vi "test TCX read (installed 71).vi"() -> ()   [LabVIEW 2011] (continued)
ers><DistanceMeters>9789.869</DistanceMeters><Cadence>71</Cadence><Extensions><TPX xmlns=\"http://www.garmin.com/xmlschemas/ActivityExtension/v2\"><Watts>262</Watts></TPX></Extensions></Trackpoint><Trackpoint><Time>2008-03-03T14:06:44Z</Time><Position><LatitudeDegrees>35.860413</LatitudeDegrees><LongitudeDegrees>-78.885609</LongitudeDegrees></Position><AltitudeMeters>95.788</AltitudeMeters><DistanceMeters>9797.562</DistanceMeters><Cadence>71</Cadence><Extensions><TPX xmlns=\"http://www.garmin.com/xmlschemas/ActivityExtension/v2\"><Watts>280</Watts></TPX></Extensions></Trackpoint><Trackpoint><Time>2008-03-03T14:06:45Z</Time><Position><LatitudeDegrees>35.860470</LatitudeDegrees><LongitudeDegrees>-78.885560</LongitudeDegrees></Position><AltitudeMeters>95.788</AltitudeMeters><DistanceMeters>9805.292</DistanceMeters><Cadence>71</Cadence><Extensions><TPX xmlns=\"http://www.garmin.com/xmlschemas/ActivityExtension/v2\"><Watts>243</Watts></TPX></Extensions></Trackpoint><Trackpoint><Time>2008-03-03T14:06:46Z</Time><Position><LatitudeDegrees>35.860528</LatitudeDegrees><LongitudeDegrees>-78.885512</LongitudeDegrees></Position><AltitudeMeters>96.269</AltitudeMeters><DistanceMeters>9813.017</DistanceMeters><Cadence>71</Cadence><Extensions><TPX xmlns=\"http://www.garmin.com/xmlschemas/ActivityExtension/v2\"><Watts>199</Watts></TPX></Extensions></Trackpoint><Trackpoint><Time>2008-03-03T14:06:47Z</Time><Position><LatitudeDegrees>35.860585</LatitudeDegrees><LongitudeDegrees>-78.885464</LongitudeDegrees></Position><AltitudeMeters>96.269</AltitudeMeters><DistanceMeters>9820.704</DistanceMeters><Cadence>71</Cadence><Extensions><TPX xmlns=\"http://www.garmin.com/xmlschemas/ActivityExtension/v2\"><Watts>198</Watts></TPX></Extensions></Trackpoint><Trackpoint><Time>2008-03-03T14:06:48Z</Time><Position><LatitudeDegrees>35.860642</LatitudeDegrees><LongitudeDegrees>-78.885415</LongitudeDegrees></Position><AltitudeMeters>96.269</AltitudeMeters><DistanceMeters>9828.424</DistanceMeters><Cadence>71</Cadence><Extensions><TPX xmlns=\"http://www.garmin.com/xmlschemas/ActivityExtension/v2\"><Watts>210</Watts></TPX></Extensions></Trackpoint><Trackpoint><Time>2008-03-03T14:06:49Z</Time><Position><LatitudeDegrees>35.860698</LatitudeDegrees><LongitudeDegrees>-78.885365</LongitudeDegrees></Position><AltitudeMeters>96.269</AltitudeMeters><DistanceMeters>9836.081</DistanceMeters><Cadence>71</Cadence><Extensions><TPX xmlns=\"http://www.garmin.com/xmlschemas/ActivityExtension/v2\"><Watts>211</Watts></TPX></Extensions></Trackpoint><Trackpoint><Time>2008-03-03T14:06:50Z</Time><Position><LatitudeDegrees>35.860754</LatitudeDegrees><LongitudeDegrees>-78.885315</LongitudeDegrees></Position><AltitudeMeters>96.269</AltitudeMeters><DistanceMeters>9843.739</DistanceMeters><Cadence>71</Cadence><Extensions><TPX xmlns=\"http://www.garmin.com/xmlschemas/ActivityExtension/v2\"><Watts>219</Watts></TPX></Extensions></Trackpoint><Trackpoint><Time>2008-03-03T14:06:51Z</Time><Position><LatitudeDegrees>35.860809</LatitudeDegrees><LongitudeDegrees>-78.885264</LongitudeDegrees></Position><AltitudeMeters>96.750</AltitudeMeters><DistanceMeters>9851.446</DistanceMeters><Cadence>71</Cadence><Extensions><TPX xmlns=\"http://www.garmin.com/xmlschemas/ActivityExtension/v2\"><Watts>217</Watts></TPX></Extensions></Trackpoint><Trackpoint><Time>2008-03-03T14:06:52Z</Time><Position><LatitudeDegrees>35.860865</LatitudeDegrees><LongitudeDegrees>-78.885214</LongitudeDegrees></Position><AltitudeMeters>97.230</AltitudeMeters><DistanceMeters>9859.071</DistanceMeters><Cadence>70</Cadence><Extensions><TPX xmlns=\"http://www.garmin.com/xmlschemas/ActivityExtension/v2\"><Watts>214</Watts></TPX></Extensions></Trackpoint><Trackpoint><Time>2008-03-03T14:06:53Z</Time><Position><LatitudeDegrees>35.860919</LatitudeDegrees><LongitudeDegrees>-78.885164</LongitudeDegrees></Position><AltitudeMeters>97.230</AltitudeMeters><DistanceMeters>9866.535</DistanceMeters><Cadence>67</Cadence><Extensions><TPX xmlns=\"http://www.garmin.com/xmlschemas/ActivityExtension/v2\"><Watts>220</Watts></TPX></Extensions></Trackpoint><Trackpoint><Time>2008-03-03T14:06:54Z</Time><Position><LatitudeDegrees>35.860975</LatitudeDegrees><LongitudeDegrees>-78.885114</LongitudeDegrees></Position><AltitudeMeters>97.230</AltitudeMeters><DistanceMeters>9874.188</DistanceMeters><Cadence>67</Cadence><Extensions><TPX xmlns=\"http://www.garmin.com/xmlschemas/ActivityExtension/v2\"><Watts>221</Watts></TPX></Extensions></Trackpoint><Trackpoint><Time>2008-03-03T14:06:55Z</Time><Position><LatitudeDegrees>35.861031</LatitudeDegrees><LongitudeDegrees>-78.885064</LongitudeDegrees></Position><AltitudeMeters>97.230</AltitudeMeters><DistanceMeters>9881.928</DistanceMeters><Cadence>69</Cadence><Extensions><TPX xmlns=\"http://www.garmin.com/xmlschemas/ActivityExtension/v2\"><Watts>245</Watts></TPX></Extensions></Trackpoint><Trackpoint><Time>2008-03-03T14:06:56Z</Time><Position><LatitudeDegrees>35.861087</LatitudeDegrees><LongitudeDegrees>-78.885015</LongitudeDegrees></Position><AltitudeMeters>96.750</AltitudeMeters><DistanceMeters>9889.609</DistanceMeters><Cadence>71</Cadence><Extensions><TPX xmlns=\"http://www.garmin.com/xmlschemas/ActivityExtension/v2\"><Watts>398</Watts></TPX></Extensions></Trackpoint><Trackpoint><Time>2008-03-03T14:06:57Z</Time><Position><LatitudeDegrees>35.861144</LatitudeDegrees><LongitudeDegrees>-78.884964</LongitudeDegrees></Position><AltitudeMeters>97.711</AltitudeMeters><DistanceMeters>9897.438</DistanceMeters><Cadence>71</Cadence><Extensions><TPX xmlns=\"http://www.garmin.com/xmlschemas/ActivityExtension/v2\"><Watts>421</Watts></TPX></Extensions></Trackpoint><Trackpoint><Time>2008-03-03T14:06:58Z</Time><Position><LatitudeDegrees>35.861201</LatitudeDegrees><LongitudeDegrees>-78.884911</LongitudeDegrees></Position><AltitudeMeters>98.192</AltitudeMeters><DistanceMeters>9905.341</DistanceMeters><Cadence>72</Cadence><Extensions><TPX xmlns=\"http://www.garmin.com/xmlschemas/ActivityExtension/v2\"><Watts>420</Watts></TPX></Extensions></Trackpoint><Trackpoint><Time>2008-03-03T14:06:59Z</Time><Position><LatitudeDegrees>35.861256</LatitudeDegrees><LongitudeDegrees>-78.884860</LongitudeDegrees></Position><AltitudeMeters>98.192</AltitudeMeters><DistanceMeters>9912.980</DistanceMeters><Cadence>71</Cadence><Extensions><TPX xmlns=\"http://www.garmin.com/xmlschemas/ActivityExtension/v2\"><Watts>419</Watts></TPX></Extensions></Trackpoint><Trackpoint><Time>2008-03-03T14:07:00Z</Time><Position><LatitudeDegrees>35.861312</LatitudeDegrees><LongitudeDegrees>-78.884809</LongitudeDegrees></Position><AltitudeMeters>98.672</AltitudeMeters><DistanceMeters>9920.728</DistanceMeters><Cadence>70</Cadence><Extensions><TPX xmlns=\"http://www.garmin.com/xmlschemas/ActivityExtension/v2\"><Watts>406</Watts></TPX></Extensions></Trackpoint><Trackpoint><Time>2008-03-03T14:07:01Z</Time><Position><LatitudeDegrees>35.861368</LatitudeDegrees><LongitudeDegrees>-78.884761</LongitudeDegrees></Position><AltitudeMeters>99.153</AltitudeMeters><DistanceMeters>9928.274</DistanceMeters><Cadence>70</Cadence><Extensions><TPX xmlns=\"http://www.garmin.com/xmlschemas/ActivityExtension/v2\"><Watts>406</Watts></TPX></Extensions></Trackpoint><Trackpoint><Time>2008-03-03T14:07:02Z</Time><Position><LatitudeDegrees>35.861424</LatitudeDegrees><LongitudeDegrees>-78.884713</LongitudeDegrees></Position><AltitudeMeters>99.634</AltitudeMeters><DistanceMeters>9935.836</DistanceMeters><Cadence>70</Cadence><Extensions><TPX xmlns=\"http://www.garmin.com/xmlschemas/ActivityExtension/v2\"><Watts>390</Watts></TPX></Extensions></Trackpoint><Trackpoint><Time>2008-03-03T14:07:03Z</Time><Position><LatitudeDegrees>35.861481</LatitudeDegrees><LongitudeDegrees>-78.884664</LongitudeDegrees></Position><AltitudeMeters>100.115</AltitudeMeters><DistanceMeters>9943.662</DistanceMeters><Cadence>69</Cadence><Extensions><TPX xmlns=\"http://www.garmin.com/xmlschemas/ActivityExtension/v2\"><Watts>387</Watts></TPX></Extensions></Trackpoint><Trackpoint><Time>2008-03-03T14:07:04Z</Time><Position><LatitudeDegrees>35.861538</LatitudeDegrees><LongitudeDegrees>-78.884615</LongitudeDegrees></Position><AltitudeMeters>100.115</AltitudeMeters><DistanceMeters>9951.247</DistanceMeters><Cadence>69</Cadence><Extensions><TPX xmlns=\"http://www.garmin.com/xmlschemas/ActivityExtension/v2\"><Watts>379</Watts></TPX></Extensions></Trackpoint><Trackpoint><Time>2008-03-03T14:07:05Z</Time><Position><LatitudeDegrees>35.861592</LatitudeDegrees><LongitudeDegrees>-78.884566</LongitudeDegrees></Position><AltitudeMeters>100.115</AltitudeMeters><DistanceMeters>9958.741</DistanceMeters><Cadence>70</Cadence><Extensions><TPX xmlns=\"http://www.garmin.com/xmlschemas/ActivityExtension/v2\"><Watts>367</Watts></TPX></Extensions></Trackpoint><Trackpoint><Time>2008-03-03T14:07:06Z</Time><Position><LatitudeDegrees>35.861647</LatitudeDegrees><LongitudeDegrees>-78.884516</LongitudeDegrees></Position><AltitudeMeters>100.595</AltitudeMeters><DistanceMeters>9966.347</DistanceMeters><Cadence>70</Cadence><Extensions><TPX xmlns=\"http://www.garmin.com/xmlschemas/ActivityExtension/v2\"><Watts>366</Watts></TPX></Extensions></Trackpoint><Trackpoint><Time>2008-03-03T14:07:07Z</Time><Position><LatitudeDegrees>35.861704</LatitudeDegrees><LongitudeDegrees>-78.884469</LongitudeDegrees></Position><AltitudeMeters>100.115</AltitudeMeters><DistanceMeters>9973.955</DistanceMeters><Cadence>72</Cadence><Extensions><TPX xmlns=\"http://www.garmin.com/xmlschemas/ActivityExtension/v2\"><Watts>375</Watts></TPX></Extensions></Trackpoint><Trackpoint><Time>2008-03-03T14:07:08Z</Time><Position><LatitudeDegrees>35.861765</LatitudeDegrees><LongitudeDegrees>-78.884424</LongitudeDegrees></Position><AltitudeMeters>100.595</AltitudeMeters><DistanceMeters>9981.838</DistanceMeters><Cadence>75</Cadence><Extensions><TPX xmlns=\"http://www.garmin.com/xmlschemas/ActivityExtension/v2\"><Watts>374</Watts></TPX></Extensions></Trackpoint><Trackpoint><Time>2008-03-03T14:07:09Z</Time><Position><LatitudeDegrees>35.861824</LatitudeDegrees><LongitudeDegrees>-78.884382</LongitudeDegrees></Position><AltitudeMeters>101.076</AltitudeMeters><DistanceMeters>9989.431</DistanceMeters><Cadence>73</Cadence><Extensions><TPX xmlns=\"http://www.garmin.com/xmlschemas/ActivityExtension/v2\"><Watts>355</Watts></TPX></Extensions></Trackpoint><Trackpoint><Time>2008-03-03T14:07:10Z</Time><Position><LatitudeDegrees>35.861884</LatitudeDegrees><LongitudeDegrees>-78.884341</LongitudeDegrees></Position><AltitudeMeters>101.076</AltitudeMeters><DistanceMeters>9997.033</DistanceMeters><Cadence>73</Cadence><Extensions><TPX xmlns=\"http://www.garmin.com/xmlschemas/ActivityExtension/v2\"><Watts>269</Watts></TPX></Extensions></Trackpoint><Trackpoint><Time>2008-03-03T14:07:11Z</Time><Position><LatitudeDegrees>35.861944</LatitudeDegrees><LongitudeDegrees>-78.884299</LongitudeDegrees></Position><AltitudeMeters>101.076</AltitudeMeters><DistanceMeters>10004.695</DistanceMeters><Cadence>73</Cadence><Extensions><TPX xmlns=\"http://www.garmin.com/xmlschemas/ActivityExtension/v2\"><Watts>270</Watts></TPX></Extensions></Trackpoint><Trackpoint><Time>2008-03-03T14:07:12Z</Time><Position><LatitudeDegrees>35.862005</LatitudeDegrees><LongitudeDegrees>-78.884257</LongitudeDegrees></Position><AltitudeMeters>101.076</AltitudeMeters><DistanceMeters>10012.445</DistanceMeters><Cadence>73</Cadence><Extensions><TPX xmlns=\"http://www.garmin.com/xmlschemas/ActivityExtension/v2\"><Watts>213</Watts></TPX></Extensions></Trackpoint><Trackpoint><Time>2008-03-03T14:07:13Z</Time><Position><LatitudeDegrees>35.862067</LatitudeDegrees><LongitudeDegrees>-78.884216</LongitudeDegrees></Position><AltitudeMeters>101.556</AltitudeMeters><DistanceMeters>10020.231</DistanceMeters><Cadence>73</Cadence><Extensions><TPX xmlns=\"http://www.garmin.com/xmlschemas/ActivityExtension/v2\"><Watts>227</Watts></TPX></Extensions></Trackpoint><Trackpoint><Time>2008-03-03T14:07:14Z</Time><Position><LatitudeDegrees>35.862130</LatitudeDegrees><LongitudeDegrees>-78.884177</LongitudeDegrees></Position><AltitudeMeters>101.556</AltitudeMeters><DistanceMeters>10028.093</DistanceMeters><Cadence>73</Cadence><Extensions><TPX xmlns=\"http://www.garmin.com/xmlschemas/ActivityExtension/v2\"><Watts>227</Watts></TPX></Extensions></Trackpoint><Trackpoint><Time>2008-03-03T14:07:15Z</Time><Position><LatitudeDegrees>35.862193</LatitudeDegrees><LongitudeDegrees>-78.884138</LongitudeDegrees></Position><AltitudeMeters>101.556</AltitudeMeters><DistanceMeters>10035.955</DistanceMeters><Cadence>73</Cadence><Extensions><TPX xmlns=\"http://www.garmin.com/xmlschemas/ActivityExtension/v2\"><Watts>222</Watts></TPX></Extensions></Trackpoint><Trackpoint><Time>2008-03-03T14:07:16Z</Time><Position><LatitudeDegrees>35.862256</LatitudeDegrees><LongitudeDegrees>-78.884100</LongitudeDegrees></Position><AltitudeMeters>102.037</AltitudeMeters><DistanceMeters>10043.738</DistanceMeters><Cadence>73</Cadence><Extensions><TPX xmlns=\"http://www.garmin.com/xmlschemas/ActivityExtension/v2\"><Watts>221</Watts></TPX></Extensions></Trackpoint><Trackpoint><Time>2008-03-03T14:07:17Z</Time><Position><LatitudeDegrees>35.862319</LatitudeDegrees><LongitudeDegrees>-78.884064</LongitudeDegrees></Position><AltitudeMeters>102.518</AltitudeMeters><DistanceMeters>10051.434</DistanceMeters><Cadence>72</Cadence><Extensions><TPX xmlns=\"http://www.garmin.com/xmlschemas/ActivityExtension/v2\"><Watts>195</Watts></TPX></Extensions></Trackpoint><Trackpoint><Time>2008-03-03T14:07:18Z</Time><Position><LatitudeDegrees>35.862383</LatitudeDegrees><LongitudeDegrees>-78.884031</LongitudeDegrees></Position><AltitudeMeters>102.518</AltitudeMeters><DistanceMeters>10059.122</DistanceMeters><Cadence>71</Cadence><Extensions><TPX xmlns=\"http://www.garmin.com/xmlschemas/ActivityExtension/v2\"><Watts>194</Watts></TPX></Extensions></Trackpoint><Trackpoint><Time>2008-03-03T14:07:19Z</Time><Position><LatitudeDegrees>35.862447</LatitudeDegrees><LongitudeDegrees>-78.883999</LongitudeDegrees></Position><AltitudeMeters>102.037</AltitudeMeters><DistanceMeters>10066.811</DistanceMeters><Cadence>72</Cadence><Extensions><TPX xmlns=\"http://www.garmin.com/xmlschemas/ActivityExtension/v2\"><Watts>227</Watts></TPX></Extensions></Trackpoint><Trackpoint><Time>2008-03-03T14:07:20Z</Time><Position><LatitudeDegrees>35.862512</LatitudeDegrees><LongitudeDegrees>-78.883969</LongitudeDegrees></Position><AltitudeMeters>102.037</AltitudeMeters><DistanceMeters>10074.514</DistanceMeters><Cadence>71</Cadence><Extensions><TPX xmlns=\"http://www.garmin.com/xmlschemas/ActivityExtension/v2\"><Watts>226</Watts></TPX></Extensions></Trackpoint><Trackpoint><Time>2008-03-03T14:07:21Z</Time><Position><LatitudeDegrees>35.862577</LatitudeDegrees><LongitudeDegrees>-78.883941</LongitudeDegrees></Position><AltitudeMeters>102.518</AltitudeMeters><DistanceMeters>10082.205</DistanceMeters><Cadence>71</Cadence><Extensions><TPX xmlns=\"http://www.garmin.com/xmlschemas/ActivityExtension/v2\"><Watts>225</Watts></TPX></Extensions></Trackpoint><Trackpoint><Time>2008-03-03T14:07:22Z</Time><Position><LatitudeDegrees>35.862643</LatitudeDegrees><LongitudeDegrees>-78.883912</LongitudeDegrees></Position><AltitudeMeters>102.518</AltitudeMeters><DistanceMeters>10089.852</DistanceMeters><Cadence>71</Cadence><Extensions><TPX xmlns=\"http://www.garmin.com/xmlschemas/ActivityExtension/v2\"><Watts>187</Watts></TPX></Extensions></Trackpoint><Trackpoint><Time>2008-03-03T14:07:23Z</Time><Position><LatitudeDegrees>35.862708</LatitudeDegrees><LongitudeDegrees>-78.883886</LongitudeDegrees></Position><AltitudeMeters>102.037</AltitudeMeters><DistanceMeters>10097.484</DistanceMeters><Cadence>71</Cadence><Extensions><TPX xmlns=\"http://www.garmin.com/xmlschemas/ActivityExtension/v2\"><Watts>189</Watts></TPX></Extensions></Trackpoint><Trackpoint><Time>2008-03-03T14:07:24Z</Time><Position><LatitudeDegrees>35.862774</LatitudeDegrees><LongitudeDegrees>-78.883861</LongitudeDegrees></Position><AltitudeMeters>102.518</AltitudeMeters><DistanceMeters>10105.122</DistanceMeters><Cadence>70</Cadence><Extensions><TPX xmlns=\"http://www.garmin.com/xmlschemas/ActivityExtension/v2\"><Watts>184</Watts></TPX></Extensions></Trackpoint><Trackpoint><Time>2008-03-03T14:07:25Z</Time><Position><LatitudeDegrees>35.862839</LatitudeDegrees><LongitudeDegrees>-78.883836</LongitudeDegrees></Position><AltitudeMeters>102.998</AltitudeMeters><DistanceMeters>10112.757</DistanceMeters><Cadence>70</Cadence><Extensions><TPX xmlns=\"http://www.garmin.com/xmlschemas/ActivityExtension/v2\"><Watts>173</Watts></TPX></Extensions></Trackpoint><Trackpoint><Time>2008-03-03T14:07:26Z</Time><Position><LatitudeDegrees>35.862905</LatitudeDegrees><LongitudeDegrees>-78.883811</LongitudeDegrees></Position><AltitudeMeters>102.518</AltitudeMeters><DistanceMeters>10120.379</DistanceMeters><Cadence>70</Cadence><Extensions><TPX xmlns=\"http://www.garmin.com/xmlschemas/ActivityExtension/v2\"><Watts>172</Watts></TPX></Extensions></Trackpoint><Trackpoint><Time>2008-03-03T14:07:27Z</Time><Position><LatitudeDegrees>35.862971</LatitudeDegrees><LongitudeDegrees>-78.883789</LongitudeDegrees></Position><AltitudeMeters>102.518</AltitudeMeters><DistanceMeters>10127.997</DistanceMeters><Cadence>70</Cadence><Extensions><TPX xmlns=\"http://www.garmin.com/xmlschemas/ActivityExtension/v2\"><Watts>151</Watts></TPX></Extensions></Trackpoint><Trackpoint><Time>2008-03-03T14:07:28Z</Time><Position><LatitudeDegrees>35.863039</LatitudeDegrees><LongitudeDegrees>-78.883771</LongitudeDegrees></Position><AltitudeMeters>102.518</AltitudeMeters><DistanceMeters>10135.639</DistanceMeters><Cadence>70</Cadence><Extensions><TPX xmlns=\"http://www.garmin.com/xmlschemas/ActivityExtension/v2\"><Watts>151</Watts></TPX></Extensions></Trackpoint><Trackpoint><Time>2008-03-03T14:07:29Z</Time><Position><LatitudeDegrees>35.863106</LatitudeDegrees><LongitudeDegrees>-78.883755</LongitudeDegrees></Position><AltitudeMeters>102.518</AltitudeMeters><DistanceMeters>10143.321</DistanceMeters><Cadence>71</Cadence><Extensions><TPX xmlns=\"http://www.garmin.com/xmlschemas/ActivityExtension/v2\"><Watts>143</Watts></TPX></Extensions></Trackpoint><Trackpoint><Time>2008-03-03T14:07:30Z</Time><Position><LatitudeDegrees>35.863175</LatitudeDegrees><LongitudeDegrees>-78.883738</LongitudeDegrees></Position><AltitudeMeters>102.518</AltitudeMeters><DistanceMeters>10151.073</DistanceMeters><Cadence>71</Cadence><Extensions><TPX xmlns=\"http://www.garmin.com/xmlschemas/ActivityExtension/v2\"><Watts>129</Watts></TPX></Extensions></Trackpoint><Trackpoint><Time>2008-03-03T14:07:31Z</Time><Position><LatitudeDegrees>35.863244</LatitudeDegrees><LongitudeDegrees>-78.883722</LongitudeDegrees></Position><AltitudeMeters>102.518</AltitudeMeters><DistanceMeters>10158.863</DistanceMeters><Cadence>71</Cadence><Extensions><TPX xmlns=\"http://www.garmin.com/xmlschemas/ActivityExtension/v2\"><Watts>127</Watts></TPX></Extensions></Trackpoint><Trackpoint><Time>2008-03-03T14:07:32Z</Time><Position><LatitudeDegrees>35.863313</LatitudeDegrees><LongitudeDegrees>-78.883706</LongitudeDegrees></Position><AltitudeMeters>102.518</AltitudeMeters><DistanceMeters>10166.655</DistanceMeters><Cadence>72</Cadence><Extensions><TPX xmlns=\"http://www.garmin.com/xmlschemas/ActivityExtension/v2\"><Watts>126</Watts></TPX></Extensions></Trackpoint><Trackpoint><Time>2008-03-03T14:07:33Z</Time><Position><LatitudeDegrees>35.863384</LatitudeDegrees><LongitudeDegrees>-78.883694</LongitudeDegrees></Position><AltitudeMeters>102.518</AltitudeMeters><DistanceMeters>10174.608</DistanceMeters><Cadence>72</Cadence><Extensions><TPX xmlns=\"http://www.garmin.com/xmlschemas/ActivityExtension/v2\"><Watts>127</Watts></TPX></Extensions></Trackpoint><Trackpoint><Time>2008-03-03T14:07:34Z</Time><Position><LatitudeDegrees>35.863456</LatitudeDegrees><LongitudeDegrees>-78.883683</LongitudeDegrees></Position><AltitudeMeters>102.518</AltitudeMeters><DistanceMeters>10182.617</DistanceMeters><Cadence>73</Cadence><Extensions><TPX xmlns=\"http://www.garmin.com/xmlschemas/ActivityExtension/v2\"><Watts>128</Watts></TPX></Extensions></Trackpoint><Trackpoint><Time>2008-03-03T14:07:35Z</Time><Position><LatitudeDegrees>35.863528</LatitudeDegrees><LongitudeDegrees>-78.883672</LongitudeDegrees></Position><AltitudeMeters>102.518</AltitudeMeters><DistanceMeters>10190.719</DistanceMeters><Cadence>74</Cadence><Extensions><TPX xmlns=\"http://www.garmin.com/xmlschemas/ActivityExtension/v2\"><Watts>129</Watts></TPX></Extensions></Trackpoint><Trackpoint><Time>2008-03-03T14:07:36Z</Time><Position><LatitudeDegrees>35.863602</LatitudeDegrees><LongitudeDegrees>-78.883661</LongitudeDegrees></Position><AltitudeMeters>102.037</AltitudeMeters><DistanceMeters>10198.949</DistanceMeters><Cadence>75</Cadence><Extensions><TPX xmlns=\"http://www.garmin.com/xmlschemas/ActivityExtension/v2\"><Watts>117</Watts></TPX></Extensions></Trackpoint><Trackpoint><Time>2008-03-03T14:07:37Z</Time><Position><LatitudeDegrees>35.863676</LatitudeDegrees><LongitudeDegrees>-78.883652</LongitudeDegrees></Position><AltitudeMeters>102.037</AltitudeMeters><DistanceMeters>10207.255</DistanceMeters><Cadence>76</Cadence><Extensions><TPX xmlns=\"http://www.garmin.com/xmlschemas/ActivityExtension/v2\"><Watts>112</Watts></TPX></Extensions></Trackpoint><Trackpoint><Time>2008-03-03T14:07:38Z</Time><Position><LatitudeDegrees>35.863751</LatitudeDegrees><LongitudeDegrees>-78.883646</LongitudeDegrees></Position><AltitudeMeters>102.037</AltitudeMeters><DistanceMeters>10215.649</DistanceMeters><Cadence>76</Cadence><Extensions><TPX xmlns=\"http://www.garmin.com/xmlschemas/ActivityExtension/v2\"><Watts>99</Watts></TPX></Extensions></Trackpoint><Trackpoint><Time>2008-03-03T14:07:39Z</Time><Position><LatitudeDegrees>35.863827</LatitudeDegrees><LongitudeDegrees>-78.883641</LongitudeDegrees></Position><AltitudeMeters>101.556</AltitudeMeters><DistanceMeters>10224.088</DistanceMeters><Cadence>77</Cadence><Extensions><TPX xmlns=\"http://www.garmin.com/xmlschemas/ActivityExtension/v2\"><Watts>90</Watts></TPX></Extensions></Trackpoint><Trackpoint><Time>2008-03-03T14:07:40Z</Time><Position><LatitudeDegrees>35.863904</LatitudeDegrees><LongitudeDegrees>-78.883636</LongitudeDegrees></Position><AltitudeMeters>101.556</AltitudeMeters><DistanceMeters>10232.604</DistanceMeters><Cadence>73</Cadence><Extensions><TPX xmlns=\"http://www.garmin.com/xmlschemas/ActivityExtension/v2\"><Watts>85</Watts></TPX></Extensions></Trackpoint><Trackpoint><Time>2008-03-03T14:07:41Z</Time><Position><LatitudeDegrees>35.863982</LatitudeDegrees><LongitudeDegrees>-78.883632</LongitudeDegrees></Position><AltitudeMeters>101.556</AltitudeMeters><DistanceMeters>10241.290</DistanceMeters><Cadence>69</Cadence><Extensions><TPX xmlns=\"http://www.garmin.com/xmlschemas/ActivityExtension/v2\"><Watts>92</Watts></TPX></Extensions></Trackpoint><Trackpoint><Time>2008-03-03T14:07:42Z</Time><Position><LatitudeDegrees>35.864060</LatitudeDegrees><LongitudeDegrees>-78.883631</LongitudeDegrees></Position><AltitudeMeters>101.556</AltitudeMeters><DistanceMeters>10249.943</DistanceMeters><Cadence>70</Cadence><Extensions><TPX xmlns=\"http://www.garmin.com/xmlschemas/ActivityExtension/v2\"><Watts>101</Watts></TPX></Extensions></Trackpoint><Trackpoint><Time>2008-03-03T14:07:43Z</Time><Position><LatitudeDegrees>35.864140</LatitudeDegrees><LongitudeDegrees>-78.883631</LongitudeDegrees></Position><AltitudeMeters>101.556</AltitudeMeters><DistanceMeters>10258.783</DistanceMeters><Cadence>72</Cadence><Extensions><TPX xmlns=\"http://www.garmin.com/xmlschemas/ActivityExtension/v2\"><Watts>91</Watts></TPX></Extensions></Trackpoint><Trackpoint><Time>2008-03-03T14:07:44Z</Time><Position><LatitudeDegrees>35.864220</LatitudeDegrees><LongitudeDegrees>-78.883633</LongitudeDegrees></Position><AltitudeMeters>101.556</AltitudeMeters><DistanceMeters>10267.762</DistanceMeters><Cadence>73</Cadence><Extensions><TPX xmlns=\"http://www.garmin.com/xmlschemas/ActivityExtension/v2\"><Watts>99</Watts></TPX></Extensions></Trackpoint><Trackpoint><Time>2008-03-03T14:07:45Z</Time><Position><LatitudeDegrees>35.864302</LatitudeDegrees><LongitudeDegrees>-78.883640</LongitudeDegrees></Position><AltitudeMeters>100.595</AltitudeMeters><DistanceMeters>10276.862</DistanceMeters><Cadence>74</Cadence><Extensions><TPX xmlns=\"http://www.garmin.com/xmlschemas/ActivityExtension/v2\"><Watts>96</Watts></TPX></Extensions></Trackpoint><Trackpoint><Time>2008-03-03T14:07:46Z</Time><Position><LatitudeDegrees>35.864385</LatitudeDegrees><LongitudeDegrees>-78.883650</LongitudeDegrees></Position><AltitudeMeters>100.595</AltitudeMeters><DistanceMeters>10286.131</DistanceMeters><Cadence>76</Cadence><Extensions><TPX xmlns=\"http://www.garmin.com/xmlschemas/ActivityExtension/v2\"><Watts>96</Watts></TPX></Extensions></Trackpoint><Trackpoint><Time>2008-03-03T14:07:47Z</Time><Position><LatitudeDegrees>35.864470</LatitudeDegrees><LongitudeDegrees>-78.883663</LongitudeDegrees></Position><AltitudeMeters>100.115</AltitudeMeters><DistanceMeters>10295.672</DistanceMeters><Cadence>77</Cadence><Extensions><TPX xmlns=\"http://www.garmin.com/xmlschemas/ActivityExtension/v2\"><Watts>87</Watts></TPX></Extensions></Trackpoint><Trackpoint><Time>2008-03-03T14:07:48Z</Time><Position><LatitudeDegrees>35.864557</LatitudeDegrees><LongitudeDegrees>-78.883678</LongitudeDegrees></Position><AltitudeMeters>100.115</AltitudeMeters><DistanceMeters>10305.455</DistanceMeters><Cadence>77</Cadence><Extensions><TPX xmlns=\"http://www.garmin.com/xmlschemas/ActivityExtension/v2\"><Watts>89</Watts></TPX></Extensions></Trackpoint><Trackpoint><Time>2008-03-03T14:07:49Z</Time><Position><LatitudeDegrees>35.864646</LatitudeDegrees><LongitudeDegrees>-78.883694</LongitudeDegrees></Position><AltitudeMeters>99.153</AltitudeMeters><DistanceMeters>10315.415</DistanceMeters><Cadence>82</Cadence><Extensions><TPX xmlns=\"http://www.garmin.com/xmlschemas/ActivityExtension/v2\"><Watts>88</Watts></TPX></Extensions></Trackpoint><Trackpoint><Time>2008-03-03T14:07:50Z</Time><Position><LatitudeDegrees>35.864737</LatitudeDegrees><LongitudeDegrees>-78.883711</LongitudeDegrees></Position><AltitudeMeters>99.153</AltitudeMeters><DistanceMeters>10325.573</DistanceMeters><Cadence>83</Cadence><Extensions><TPX xmlns=\"http://www.garmin.com/xmlschemas/ActivityExtension/v2\"><Watts>94</Watts></TPX></Extensions></Trackpoint><Trackpoint><Time>2008-03-03T14:07:51Z</Time><Position><LatitudeDegrees>35.864828</LatitudeDegrees><LongitudeDegrees>-78.883731</LongitudeDegrees></Position><AltitudeMeters>98.672</AltitudeMeters><DistanceMeters>10335.891</DistanceMeters><Cadence>83</Cadence><Extensions><TPX xmlns=\"http://www.garmin.com/xmlschemas/ActivityExtension/v2\"><Watts>93</Watts></TPX></Extensions></Trackpoint><Trackpoint><Time>2008-03-03T14:07:52Z</Time><Position><LatitudeDegrees>35.864920</LatitudeDegrees><LongitudeDegrees>-78.883754</LongitudeDegrees></Position><AltitudeMeters>98.192</AltitudeMeters><DistanceMeters>10346.277</DistanceMeters><Cadence>85</Cadence><Extensions><TPX xmlns=\"http://www.garmin.com/xmlschemas/ActivityExtension/v2\"><Watts>80</Watts></TPX></Extensions></Trackpoint><Trackpoint><Time>2008-03-03T14:07:53Z</Time><Position><LatitudeDegrees>35.865011</LatitudeDegrees><LongitudeDegrees>-78.883780</LongitudeDegrees></Position><AltitudeMeters>98.672</AltitudeMeters><DistanceMeters>10356.652</DistanceMeters><Cadence>85</Cadence><Extensions><TPX xmlns=\"http://www.garmin.com/xmlschemas/ActivityExtension/v2\"><Watts>79</Watts></TPX></Extensions></Trackpoint><Trackpoint><Time>2008-03-03T14:07:54Z</Time><Position><LatitudeDegrees>35.865105</LatitudeDegrees><LongitudeDegrees>-78.883795</LongitudeDegrees></Position><AltitudeMeters>98.672</AltitudeMeters><DistanceMeters>10367.121</DistanceMeters><Cadence>86</Cadence><Extensions><TPX xmlns=\"http://www.garmin.com/xmlschemas/ActivityExtension/v2\"><Watts>104</Watts></TPX></Extensions></Trackpoint><Trackpoint><Time>2008-03-03T14:07:55Z</Time><Position><LatitudeDegrees>35.865197</LatitudeDegrees><LongitudeDegrees>-78.883784</LongitudeDegrees></Position><AltitudeMeters>98.192</AltitudeMeters><DistanceMeters>10377.354</DistanceMeters><Cadence>86</Cadence><Extensions><TPX xmlns=\"http://www.garmin.com/xmlschemas/ActivityExtension/v2\"><Watts>119</Watts></TPX></Extensions></Trackpoint><Trackpoint><Time>2008-03-03T14:07:56Z</Time><Position><LatitudeDegrees>35.865279</LatitudeDegrees><LongitudeDegrees>-78.883729</LongitudeDegrees></Position><AltitudeMeters>98.672</AltitudeMeters><DistanceMeters>10387.548</DistanceMeters><Cadence>85</Cadence><Extensions><TPX xmlns=\"http://www.garmin.com/xmlschemas/ActivityExtension/v2\"><Watts>131</Watts></TPX></Extensions></Trackpoint><Trackpoint><Time>2008-03-03T14:07:57Z</Time><Position><LatitudeDegrees>35.865332</LatitudeDegrees><LongitudeDegrees>-78.883639</LongitudeDegrees></Position><AltitudeMeters>98.672</AltitudeMeters><DistanceMeters>10397.631</DistanceMeters><Cadence>81</Cadence><Extensions><TPX xmlns=\"http://www.garmin.com/xmlschemas/ActivityExtension/v2\"><Watts>139</Watts></TPX></Extensions></Trackpoint><Trackpoint><Time>2008-03-03T14:07:58Z</Time><Position><LatitudeDegrees>35.865370</LatitudeDegrees><LongitudeDegrees>-78.883534</LongitudeDegrees></Position><AltitudeMeters>98.672</AltitudeMeters><DistanceMeters>10408.059</DistanceMeters><Cadence>81</Cadence><Extensions><TPX xmlns=\"http://www.garmin.com/xmlschemas/ActivityExtension/v2\"><Watts>136</Watts></TPX></Extensions></Trackpoint><Trackpoint><Time>2008-03-03T14:07:59Z</Time><Position><LatitudeDegrees>35.865390</LatitudeDegrees><LongitudeDegrees>-78.883427</LongitudeDegrees></Position><AltitudeMeters>99.153</AltitudeMeters><DistanceMeters>10417.958</DistanceMeters><Cadence>84</Cadence><Extensions><TPX xmlns=\"http://www.garmin.com/xmlschemas/ActivityExtension/v2\"><Watts>167</Watts></TPX></Extensions></Trackpoint><Trackpoint><Time>2008-03-03T14:08:00Z</Time><Position><LatitudeDegrees>35.865400</LatitudeDegrees><LongitudeDegrees>-78.883325</LongitudeDegrees></Position><AltitudeMeters>99.153</AltitudeMeters><DistanceMeters>10427.103</DistanceMeters><Cadence>84</Cadence><Extensions><TPX xmlns=\"http://www.garmin.com/xmlschemas/ActivityExtension/v2\"><Watts>165</Watts></TPX></Extensions></Trackpoint><Trackpoint><Time>2008-03-03T14:08:01Z</Time><Position><LatitudeDegrees>35.865416</LatitudeDegrees><LongitudeDegrees>-78.883217</LongitudeDegrees></Position><AltitudeMeters>99.153</AltitudeMeters><DistanceMeters>10437.022</DistanceMeters><Cadence>83</Cadence><Extensions><TPX xmlns=\"http://www.garmin.com/xmlschemas/ActivityExtension/v2\"><Watts>313</Watts></TPX></Extensions></Trackpoint><Trackpoint><Time>2008-03-03T14:08:02Z</Time><Position><LatitudeDegrees>35.865430</LatitudeDegrees><LongitudeDegrees>-78.883121</LongitudeDegrees></Position><AltitudeMeters>99.634</AltitudeMeters><DistanceMeters>10445.831</DistanceMeters><Cadence>84</Cadence><Extensions><TPX xmlns=\"http://www.garmin.com/xmlschemas/ActivityExtension/v2\"><Watts>511</Watts></TPX></Extensions></Trackpoint><Trackpoint><Time>2008-03-03T14:08:03Z</Time><Position><LatitudeDegrees>35.865451</LatitudeDegrees><LongitudeDegrees>-78.883018</LongitudeDegrees></Position><AltitudeMeters>100.115</AltitudeMeters><DistanceMeters>10455.514</DistanceMeters><Cadence>84</Cadence><Extensions><TPX xmlns=\"http://www.garmin.com/xmlschemas/ActivityExtension/v2\"><Watts>508</Watts></TPX></Extensions></Trackpoint><Trackpoint><Time>2008-03-03T14:08:04Z</Time><Position><LatitudeDegrees>35.865474</LatitudeDegrees><LongitudeDegrees>-78.882915</LongitudeDegrees></Position><AltitudeMeters>100.595</AltitudeMeters><DistanceMeters>10465.014</DistanceMeters><Cadence>89</Cadence><Extensions><TPX xmlns=\"http://www.garmin.com/xmlschemas/ActivityExtension/v2\"><Watts>643</Watts></TPX></Extensions></Trackpoint><Trackpoint><Time>2008-03-03T14:08:05Z</Time><Position><LatitudeDegrees>35.865497</LatitudeDegrees><LongitudeDegrees>-78.882812</LongitudeDegrees></Position><AltitudeMeters>100.595</AltitudeMeters><DistanceMeters>10474.699</DistanceMeters><Cadence>90</Cadence><Extensions><TPX xmlns=\"http://www.garmin.com/xmlschemas/ActivityExtension/v2\"><Watts>643</Watts></TPX></Extensions></Trackpoint><Trackpoint><Time>2008-03-03T14:08:06Z</Time><Position><LatitudeDegrees>35.865523</LatitudeDegrees><LongitudeDegrees>-78.882709</LongitudeDegrees></Position><AltitudeMeters>101.076</AltitudeMeters><DistanceMeters>10484.491</DistanceMeters><Cadence>93</Cadence><Extensions><TPX xmlns=\"http://www.garmin.com/xmlschemas/ActivityExtension/v2\"><Watts>630</Watts></TPX></Extensions></Trackpoint><Trackpoint><Time>2008-03-03T14:08:07Z</Time><Position><LatitudeDegrees>35.865550</LatitudeDegrees><LongitudeDegrees>-78.882602</LongitudeDegrees></Position><AltitudeMeters>101.076</AltitudeMeters><DistanceMeters>10494.531</DistanceMeters><Cadence>97</Cadence><Extensions><TPX xmlns=\"http://www.garmin.com/xmlschemas/ActivityExtension/v2\"><Watts>641</Watts></TPX></Extensions></Trackpoint><Trackpoint><Time>2008-03-03T14:08:08Z</Time><Position><LatitudeDegrees>35.865579</LatitudeDegrees><LongitudeDegrees>-78.882495</LongitudeDegrees></Position><AltitudeMeters>101.076</AltitudeMeters><DistanceMeters>10504.790</DistanceMeters><Cadence>101</Cadence><Extensions><TPX xmlns=\"http://www.garmin.com/xmlschemas/ActivityExtension/v2\"><Watts>635</Watts></TPX></Extensions></Trackpoint><Trackpoint><Time>2008-03-03T14:08:09Z</Time><Position><LatitudeDegrees>35.865612</LatitudeDegrees><LongitudeDegrees>-78.882387</LongitudeDegrees></Position><AltitudeMeters>101.556</AltitudeMeters><DistanceMeters>10515.158</DistanceMeters><Cadence>96</Cadence><Extensions><TPX xmlns=\"http://www.garmin.com/xmlschemas/ActivityExtension/v2\"><Watts>381</Watts></TPX></Extensions></Trackpoint><Trackpoint><Time>2008-03-03T14:08:10Z</Time><Position><LatitudeDegrees>35.865647</LatitudeDegrees><LongitudeDegrees>-78.882282</LongitudeDegrees></Position><AltitudeMeters>101.076</AltitudeMeters><DistanceMeters>10525.426</DistanceMeters><Cadence>96</Cadence><Extensions><TPX xmlns=\"http://www.garmin.com/xmlschemas/ActivityExtension/v2\"><Watts>379</Watts></TPX></Extensions></Trackpoint><Trackpoint><Time>2008-03-03T14:08:11Z</Time><Position><LatitudeDegrees>35.865684</LatitudeDegrees><LongitudeDegrees>-78.882179</LongitudeDegrees></Position><AltitudeMeters>101.556</AltitudeMeters><DistanceMeters>10535.594</DistanceMeters><Cadence>83</Cadence><Extensions><TPX xmlns=\"http://www.garmin.com/xmlschemas/ActivityExtension/v2\"><Watts>155</Watts></TPX></Extensions></Trackpoint><Trackpoint><Time>2008-03-03T14:08:12Z</Time><Position><LatitudeDegrees>35.865723</LatitudeDegrees><LongitudeDegrees>-78.882077</LongitudeDegrees></Position><AltitudeMeters>101.556</AltitudeMeters><DistanceMeters>10545.769</DistanceMeters><Cadence>83</Cadence><Extensions><TPX xmlns=\"http://www.garmin.com/xmlschemas/ActivityExtension/v2\"><Watts>155</Watts></TPX></Extensions></Trackpoint><Trackpoint><Time>2008-03-03T14:08:13Z</Time><Position><LatitudeDegrees>35.865764</LatitudeDegrees><LongitudeDegrees>-78.881976</LongitudeDegrees></Position><AltitudeMeters>101.556</AltitudeMeters><DistanceMeters>10555.979</DistanceMeters><Cadence>83</Cadence><Extensions><TPX xmlns=\"http://www.garmin.com/xmlschemas/ActivityExtension/v2\"><Watts>150</Watts></TPX></Extensions></Trackpoint><Trackpoint><Time>2008-03-03T14:08:14Z</Time><Position><LatitudeDegrees>35.865805</LatitudeDegrees><LongitudeDegrees>-78.881874</LongitudeDegrees></Position><AltitudeMeters>101.076</AltitudeMeters><DistanceMeters>10566.254</DistanceMeters><Cadence>83</Cadence><Extensions><TPX xmlns=\"http://www.garmin.com/xmlschemas/ActivityExtension/v2\"><Watts>154</Watts></TPX></Extensions></Trackpoint><Trackpoint><Time>2008-03-03T14:08:15Z</Time><Position><LatitudeDegrees>35.865845</LatitudeDegrees><LongitudeDegrees>-78.881772</LongitudeDegrees></Position><AltitudeMeters>101.076</AltitudeMeters><DistanceMeters>10576.470</DistanceMeters><Cadence>83</Cadence><Extensions><TPX xmlns=\"http://www.garmin.com/xmlschemas/ActivityExtension/v2\"><Watts>151</Watts></TPX></Extensions></Trackpoint><Trackpoint><Time>2008-03-03T14:08:16Z</Time><Position><LatitudeDegrees>35.865884</LatitudeDegrees><LongitudeDegrees>-78.881670</LongitudeDegrees></Position><AltitudeMeters>100.595</AltitudeMeters><DistanceMeters>10586.667</DistanceMeters><Cadence>84</Cadence><Extensions><TPX xmlns=\"http://www.garmin.com/xmlschemas/ActivityExtension/v2\"><Watts>153</Watts></TPX></Extensions></Trackpoint><Trackpoint><Time>2008-03-03T14:08:17Z</Time><Position><LatitudeDegrees>35.865924</LatitudeDegrees><LongitudeDegrees>-78.881566</LongitudeDegrees></Position><AltitudeMeters>101.076</AltitudeMeters><DistanceMeters>10597.042</DistanceMeters><Cadence>85</Cadence><Extensions><TPX xmlns=\"http://www.garmin.com/xmlschemas/ActivityExtension/v2\"><Watts>142</Watts></TPX></Extensions></Trackpoint><Trackpoint><Time>2008-03-03T14:08:18Z</Time><Position><LatitudeDegrees>35.865966</LatitudeDegrees><LongitudeDegrees>-78.881461</LongitudeDegrees></Position><AltitudeMeters>100.595</AltitudeMeters><DistanceMeters>10607.634</DistanceMeters><Cadence>86</Cadence><Extensions><TPX xmlns=\"http://www.garmin.com/xmlschemas/ActivityExtension/v2\"><Watts>134</Watts></TPX></Extensions></Trackpoint><Trackpoint><Time>2008-03-03T14:08:19Z</Time><Position><LatitudeDegrees>35.866009</LatitudeDegrees><LongitudeDegrees>-78.881355</LongitudeDegrees></Position><AltitudeMeters>100.115</AltitudeMeters><DistanceMeters>10618.303</DistanceMeters><Cadence>88</Cadence><Extensions><TPX xmlns=\"http://www.garmin.com/xmlschemas/ActivityExtension/v2\"><Watts>134</Watts></TPX></Extensions></Trackpoint><Trackpoint><Time>2008-03-03T14:08:20Z</Time><Position><LatitudeDegrees>35.866053</LatitudeDegrees><LongitudeDegrees>-78.881249</LongitudeDegrees></Position><AltitudeMeters>100.115</AltitudeMeters><DistanceMeters>10629.075</DistanceMeters><Cadence>88</Cadence><Extensions><TPX xmlns=\"http://www.garmin.com/xmlschemas/ActivityExtension/v2\"><Watts>135</Watts></TPX></Extensions></Trackpoint><Trackpoint><Time>2008-03-03T14:08:21Z</Time><Position><LatitudeDegrees>35.866097</LatitudeDegrees><LongitudeDegrees>-78.881141</LongitudeDegrees></Position><AltitudeMeters>99.634</AltitudeMeters><DistanceMeters>10640.002</DistanceMeters><Cadence>89</Cadence><Extensions><TPX xmlns=\"http://www.garmin.com/xmlschemas/ActivityExtension/v2\"><Watts>139</Watts></TPX></Extensions></Trackpoint><Trackpoint><Time>2008-03-03T14:08:22Z</Time><Position><LatitudeDegrees>35.866143</LatitudeDegrees><LongitudeDegrees>-78.881034</LongitudeDegrees></Position><AltitudeMeters>99.634</AltitudeMeters><DistanceMeters>10650.905</DistanceMeters><Cadence>89</Cadence><Extensions><TPX xmlns=\"http://www.garmin.com/xmlschemas/ActivityExtension/v2\"><Watts>139</Watts></TPX></Extensions></Trackpoint><Trackpoint><Time>2008-03-03T14:08:23Z</Time><Position><LatitudeDegrees>35.866187</LatitudeDegrees><LongitudeDegrees>-78.880927</LongitudeDegrees></Position><AltitudeMeters>100.115</AltitudeMeters><DistanceMeters>10661.752</DistanceMeters><Cadence>88</Cadence><Extensions><TPX xmlns=\"http://www.garmin.com/xmlschemas/ActivityExtension/v2\"><Watts>145</Watts></TPX></Extensions></Trackpoint><Trackpoint><Time>2008-03-03T14:08:24Z</Time><Position><LatitudeDegrees>35.866231</LatitudeDegrees><LongitudeDegrees>-78.880820</LongitudeDegrees></Position><AltitudeMeters>99.634</AltitudeMeters><DistanceMeters>10672.553</DistanceMeters><Cadence>87</Cadence><Extensions><TPX xmlns=\"http://www.garmin.com/xmlschemas/ActivityExtension/v2\"><Watts>146</Watts></TPX></Extensions></Trackpoint><Trackpoint><Time>2008-03-03T14:08:25Z</Time><Position><LatitudeDegrees>35.866273</LatitudeDegrees><LongitudeDegrees>-78.880715</LongitudeDegrees></Position><AltitudeMeters>99.153</AltitudeMeters><DistanceMeters>10683.120</DistanceMeters><Cadence>85</Cadence><Extensions><TPX xmlns=\"http://www.garmin.com/xmlschemas/ActivityExtension/v2\"><Watts>142</Watts></TPX></Extensions></Trackpoint
